vi "释放通讯信号量.vi"(8 "error in (no error)":errorcluster) -> (0 "error out":errorcluster)   [LabVIEW 2016, in "斯坦道总氮.lvlib"]
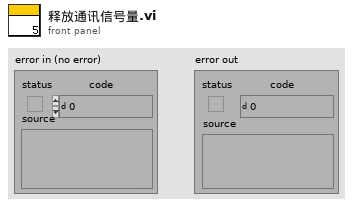
[diagram p1: front panel]
types:
  T1 = typedef "Semaphore RefNum" = refnum<k1>
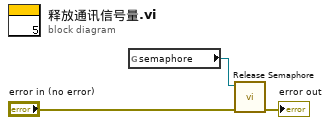
[diagram p0: block diagram]
diagram:
  n1 = global read "VAR总磷总氮全局变量.vi" "semaphore"() -> (w3:T1)
  n2 = call <vilib>:"Release Semaphore.vi"("error in (no error)"="error in (no error)", "semaphore"=w3) -> ("error out"=→"error out":errorcluster)  [unwired: 4 in, 1 out]
